vi "AccelToVib.vi"(8 "error in (no error)":errorcluster, 9 "Filters":T1={"LP Passband"=1300.0, "HP Stopband"=300.0, "LP Stopband"=1400.0, "HP Passband"=250.0} {"HP Passband" min=1.0 step=1.0 format="%#.4f"; "LP Stopband" min=1.0 step=1.0 format="%#.4f"; "HP Stopband" min=1.0 step=1.0 format="%#.4f"; "LP Passband" min=1.0 step=1.0 format="%#.4f"}, 10 "Waveform":waveform(dbl), 11 "mV/(m/s2)":dbl) -> (0 "error out":errorcluster, 3 "VP_VR_AP_AR":dbl[](array[numeric]))   [LabVIEW 2018, in "Vibration.lvlib"]
uses:
  Vibration.lvlib
  Modules/Testing UI 3/Private Controls/Cutoff Frequency.ctl
  <vilib>/addons/_NISVFA/_Shared subVIs/Controls/svc_Engineering Units Text Ring.ctl
  <vilib>/addons/_NISVFA/_Shared subVIs/Controls/svc_Channel Info.ctl
  <vilib>/addons/_NISVFA/_Shared subVIs/Controls/svc_Weighting Filter Text Ring.ctl
  <vilib>/addons/Sound and Vibration/svt_Calibration/SVL Scale Voltage to EU (1 Ch).vi
  <vilib>/addons/_NISVFA/_Shared subVIs/Common/svc_Set SV Channel Info.vi
  <vilib>/addons/_NISVFA/_Shared subVIs/Common/svc_Set SV Channel Info (variant).vi
  <vilib>/addons/_NISVFA/_Shared subVIs/Common/SVL Set dB Reference (variant).vi
  <vilib>/addons/Sound and Vibration/svt_Level/SVL Peak Level (1 Ch).vi
  <vilib>/addons/Sound and Vibration/svt_Level/SVL RMS Level (1 Ch).vi
  <vilib>/addons/Sound and Vibration/svt_Integration/SVL Integration (1 Ch).vi
  <vilib>/addons/Sound and Vibration/Order Analysis/Referece Data Processing/OAT FIR Preprocess Filter (1 Channel).vi
  <vilib>/addons/_NISVFA/_Shared subVIs/Common/svc_Caller VI Returned in Error Source.vi
  <vilib>/addons/_NISVFA/_Shared subVIs/Common/svc_Engineering Units to Unit Label.vi
  <vilib>/addons/_NISVFA/_Shared subVIs/Common/svc_Set dB ref if Pascal.vi
  <vilib>/addons/_NISVFA/_Shared subVIs/Common/svc_Compute Scale Factor to Convert C to EU.vi
  <vilib>/addons/_NISVFA/_Shared subVIs/Common/svc_Compute Scale Factor to Convert V to EU.vi
  <vilib>/addons/Sound and Vibration/svt_Level/SoundVib_VibrationLevel.lvlib
  <vilib>/addons/Sound and Vibration/svt_Integration/SoundVib_Integration.lvlib
  <vilib>/addons/Sound and Vibration/svt_Calibration/SoundVib_Calibration.lvlib
  <vilib>/addons/Sound and Vibration/Order Analysis/Referece Data Processing/SoundVib_RefDataProcess.lvlib
  Modules/Testing UI 3/Testing UI 3.lvlib
panel:
  # "VI Property set to Inline. Clone Memory"
  # "Highpass Cutoff Frequency"
  # "Lowpass Cutoff Frequency"
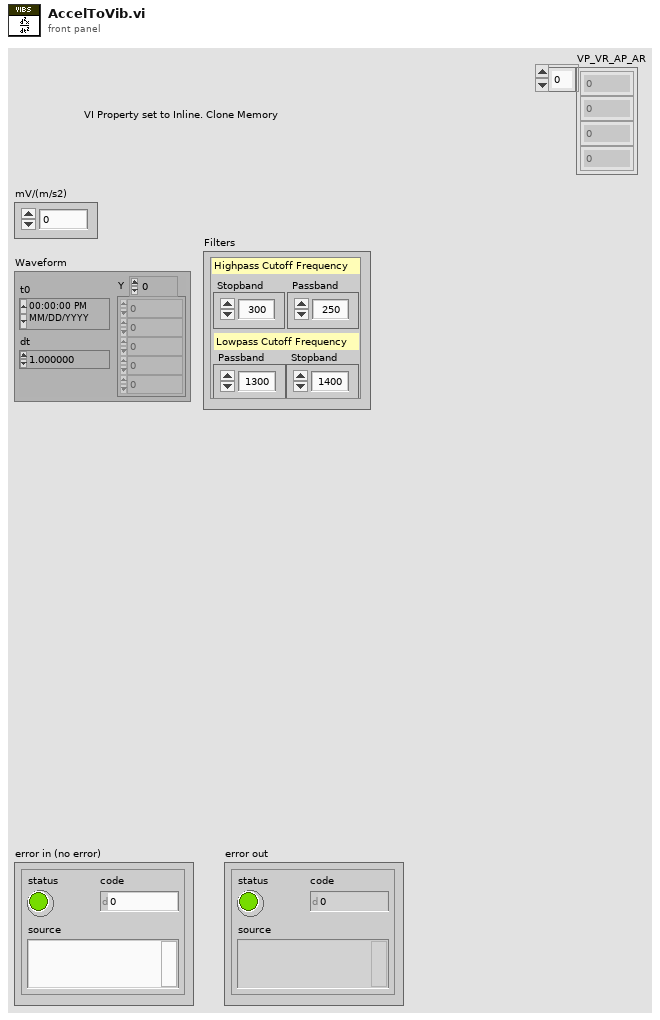
[diagram p1: front panel]
types:
  T1 = typedef "Testing UI 3.lvlib/Cutoff Frequency.ctl" = cluster{"LP Passband":dbl, "HP Stopband":dbl, "LP Stopband":dbl, "HP Passband":dbl}
  T2 = typedef "svc_Channel Info.ctl" = cluster{"sensor sensitivity":dbl, "engineering units":T3, "dB reference":dbl, "custom label":string, "weighting filter":T4, "pregain":dbl}
  T3 = typedef "svc_Engineering Units Text Ring.ctl" = u16
  T4 = typedef "svc_Weighting Filter Text Ring.ctl" = u16
  T5 = cluster{"fpass 1":dbl, "fstop 1":dbl, "fpass 2":dbl, "fstop 2":dbl}
  T6 = enum32{"Lowpass", "Highpass", "Bandpass", "Bandstop"}
  T7 = enum16{"single integration", "double integration"}
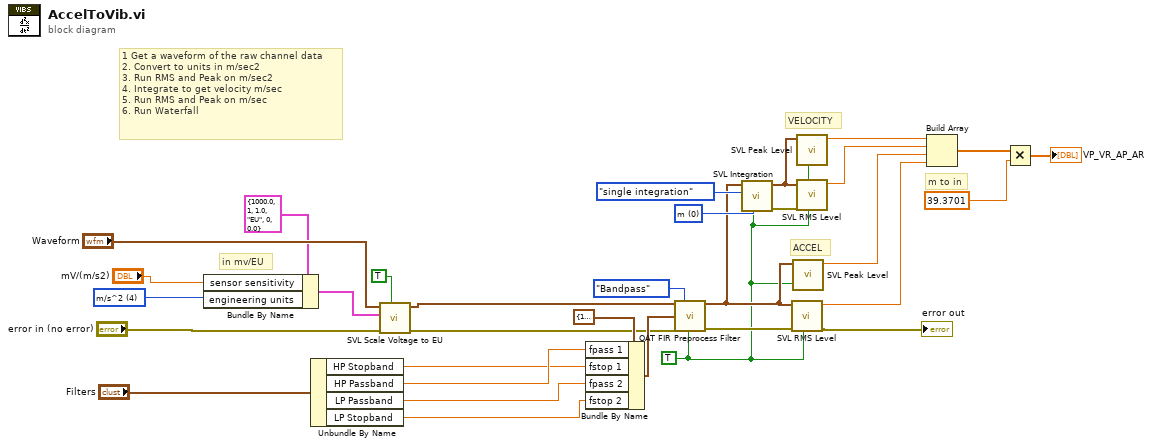
[diagram p0: block diagram]
diagram:
  w11 = TRUE ("restart")
  w15 = T3 4 items=["custom..."=0, "V"=1, "A"=21, "Pa"=2, "N"=20, "g"=3, "m/s^2"=4, "m/s"=5, "m"=6, "mm/s"=12, "mm"=13, "micron/s"=14, "micron"=15, "in/s^2"=7, "in/s"=8, "in"=9, "mil/s"=10, "mil"=11, "rad/s^2"=16, "rad/s"=17, "rad"=18, "deg/s^2"=26, "deg/s"=27, "deg"=28, "RPM"=22, "cycle/s^2"=23, "Hz"=24, "cycle"=25, "strain"=19] ("engineering units")
  w23 = 0 items=["no change"=-1, "m"=0, "mm"=2, "microns"=3, "in"=1, "mils"=5] ("length units")
  # "in mv/EU"
  # "m to in"
  # "VELOCITY"
  # "ACCEL"
  # "1 Get a waveform of the raw channel data\n2. Convert to units in m/sec2\n3. Run RMS and Peak on m/sec2\n4. Integrate to get velocity m/sec\n5. Run RMS and Peak on m/sec\n6. Run Waterfall"
  n1 = Bundle By Name(cluster=T2 {"sensor sensitivity"=1000.0, "engineering units"=1, "dB reference"=1.0, "custom label"="EU", "weighting filter"=0, "pregain"=0.0} ("channel info"), "sensor sensitivity"="mV/(m/s2)", "engineering units"=w15) -> (w16:T2)
  n2 = Unbundle By Name("Filters") -> ("HP Stopband"=w21:dbl, "HP Passband"=w31:dbl, "LP Passband"=w27:dbl, "LP Stopband"=w32:dbl)
  n3 = call-poly <vilib>:"SVL Scale Voltage to EU.vi"("write waveform attributes? (T)"=TRUE, "error in (no error)"="error in (no error)", "channel info"=w16, "signal [V]"="Waveform") -> ("error out"=w9:errorcluster, "scaled signal [EU]"=w12:waveform(dbl))  [unwired: 5 in, 1 out]
  n4 = Bundle By Name(cluster=T5 {"fpass 1"=100.0, "fstop 1"=200.0, "fpass 2"=0.0, "fstop 2"=0.0} ("freq specs [Hz]"), "fpass 1"=w31, "fstop 1"=w21, "fpass 2"=w27, "fstop 2"=w32) -> (w20:T5)
  n5 = call-poly <vilib>:"OAT FIR Preprocess Filter.vi"("scaled signal [EU]"=w12, "filter type"=T6."Bandpass", "reset? (F)"=w11, "freq specs [Hz]"=w20, "error in (no error)"=w9) -> ("filtered scaled signal [EU]"=w13:waveform(dbl), "error out"=w30:errorcluster)  [unwired: 8 in, 1 out]
  n6 = call-poly <vilib>:"SVL Integration.vi"("reset filter (F)"=w11, "length units"=w23, "integration type"=T7."single integration", "scaled signal [EU]"=w13) -> ("error out"=w24:errorcluster, "integrated signal"=w25:waveform(dbl))  [unwired: 5 in, 1 out]
  n7 = call-poly <vilib>:"SVL RMS Level.vi"("restart averaging (F)"=w11, "error in (no error)"=w30, "scaled signal [EU]"=w13) -> ("error out"=→"error out":errorcluster, "RMS level [EU rms]"=w4:dbl)  [unwired: 6 in, 1 out]
  n8 = call-poly <vilib>:"SVL Peak Level.vi"("restart averaging (F)"=w11, "scaled signal [EU]"=w13) -> ("peak level [EU]"=w5:dbl)  [unwired: 7 in, 2 out]
  n9 = call-poly <vilib>:"SVL Peak Level.vi"("restart averaging (F)"=w11, "scaled signal [EU]"=w25) -> ("peak level [EU]"=w7:dbl)  [unwired: 7 in, 2 out]
  n10 = call-poly <vilib>:"SVL RMS Level.vi"("restart averaging (F)"=w11, "error in (no error)"=w24, "scaled signal [EU]"=w25) -> ("RMS level [EU rms]"=w6:dbl)  [unwired: 6 in, 2 out]
  n11 = Build Array(w7, w6, w5, w4) -> (w3:dbl[])
  n12 = Multiply(x=w3, y=39.3701) -> (x*y=→"VP_VR_AP_AR":dbl[])
